vi "ex4.vi"() -> ()   [LabVIEW 2019]
panel:
  out "led 1":bool
  in  "bp1":bool
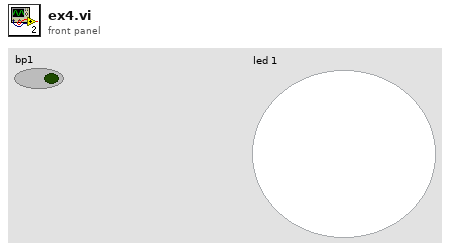
[diagram p1: front panel]
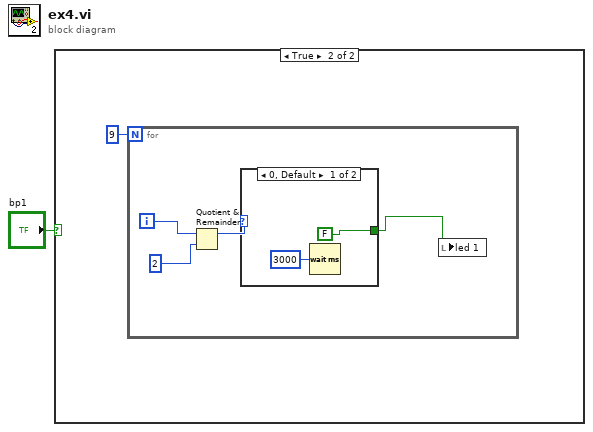
[diagram p0: block diagram]
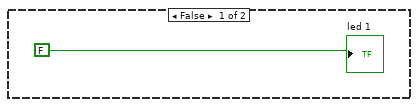
[diagram p2: hidden frame]
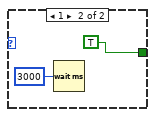
[diagram p3: hidden frame]
diagram:
  n1 = case shown="True" "bp1" {
    frame False {
      "led 1" <- FALSE
    }
    frame True {
      n2 = for {
        N: 9 -> [_]
        i -> [w6]
        n3 = Quotient & Remainder(x=w6, y=2) -> (x-y*floor(x/y)=w7:i32)  [unwired: 1 out]
        n4 = case shown="0, Default" w7 {
          tunnel: [FALSE TRUE] -> w4
          frame 0, Default {
            n5 = Wait (ms)(milliseconds to wait=u32 3000) -> ()  [unwired: 1 out]
          }
          frame 1 {
            n6 = Wait (ms)(milliseconds to wait=u32 3000) -> ()  [unwired: 1 out]
          }
        }
        n7 = local write "led 1"(w4) -> ()
      }
    }
  }
